vi "Validate Main Time.vi"(0 "Main time":u16) -> (2 "Main Time":u16, 3 "Warning":string, 4 "Frequency (Hz)":dbl)   [LabVIEW 2019]
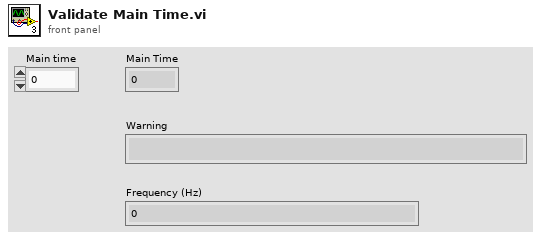
[diagram p1: front panel]
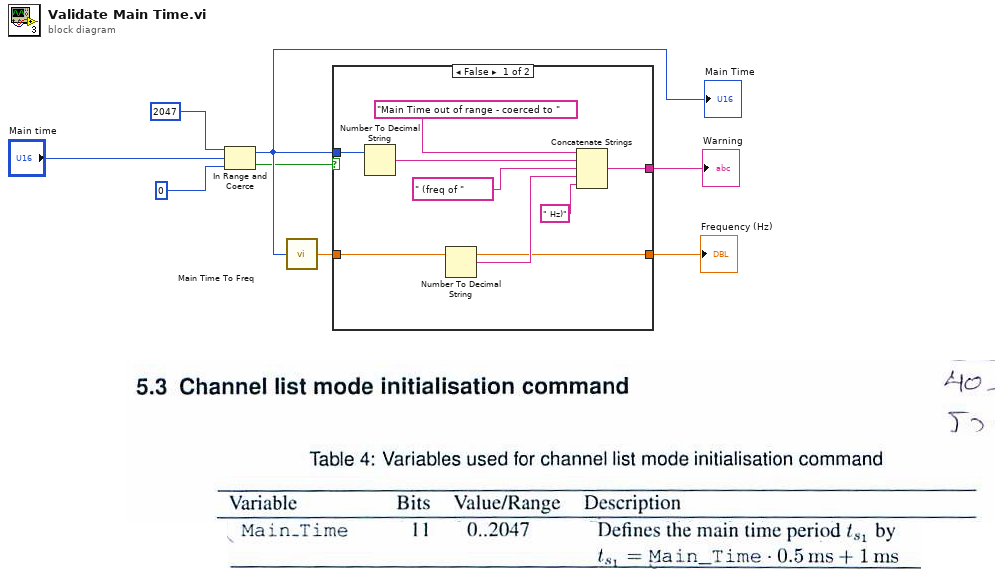
[diagram p0: block diagram]
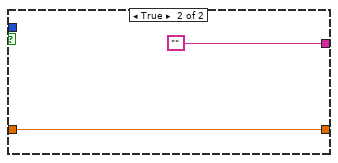
[diagram p2: hidden frame]
diagram:
  n1 = In Range and Coerce(upper limit=u16 2047, x="Main time", lower limit=u16 0) -> (coerced(x)=w6:u16, In Range?=w4:bool)
  "Main Time" <- w6
  n2 = call "Main Time To Freq.vi"("Main Time"=w6) -> ("Frequency (Hz)"=w7:dbl)
  n3 = case shown="False" w4 {
    tunnel: w6 -> [w13 _]
    tunnel: [w14 ""] -> w5
    tunnel: w7 -> [w9 w17]
    tunnel: [w9 w17] -> w8
    frame False {
      n4 = Number To Decimal String(number=w13) -> (decimal integer string=w15:string)  [unwired: 1 in]
      n5 = Number To Decimal String(number=w9) -> (decimal integer string=w11:string)  [unwired: 1 in]
      n6 = Concatenate Strings("Main Time out of range - coerced to ", w15, " (freq of " ("string"), w11, " Hz)" ("string")) -> (w14:string)
    }
    frame True {
    }
  }
  "Frequency (Hz)" <- w8
  "Warning" <- w5
